vi "Display name.vi"(1 "State In":T1) -> (0 "Name":string)   [LabVIEW 2018, in "ArrayDimension.xnode"]
uses:
  ArrayDimension.xnode
  State.ctl
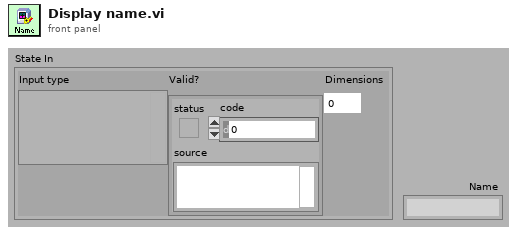
[diagram p1: front panel]
types:
  T1 = typedef "ArrayDimension.xnode/State.ctl" = cluster{"Input type":variant, "Valid?":errorcluster, "Dimensions":i32}
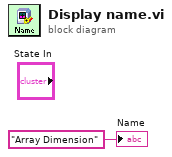
[diagram p0: block diagram]
diagram:
  "Name" <- "Array Dimension" ("Name")
